vi "AlliGator Get Image Smoothing String.vi"(8 "Error In":errorcluster, 11 "Image Binning Options":T1 {"Bin" min=1}) -> (0 "Error Out":errorcluster, 3 "String":string)   [LabVIEW 2021, in "AlliGator Source Image.lvlib"]
doc: "Builds image smoothing options string."
uses:
  AlliGator Image Smoothing Options.ctl
  Arrays/Kernel Type.ctl
  Arrays/Smoothing Algorithm.ctl
  AlliGator Source Image.lvlib
  Arrays/Arrays.lvlib
  AlliGator Settings.lvlib
panel:
  # "see the AlliGator License on the block diagram (Ctrl+E or Window:Show Block Diagram)"
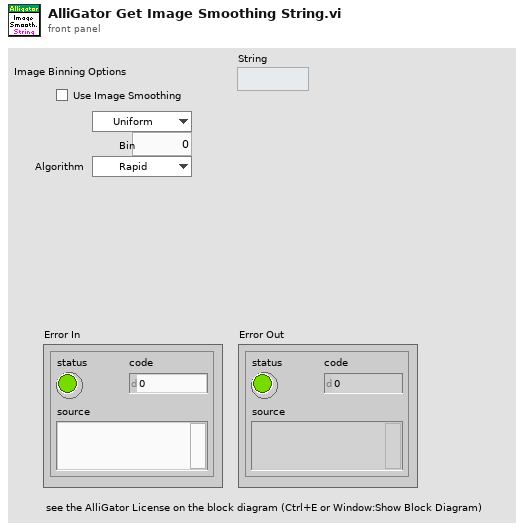
[diagram p1: front panel]
types:
  T1 = typedef "AlliGator Settings.lvlib/AlliGator Image Smoothing Options.ctl" = cluster{"Use Image Smoothing":bool, "Kernel Type":T2, "Bin":i32, "Algorithm":T3}
  T2 = typedef "Arrays.lvlib/Kernel Type.ctl" = enum16{"Uniform", "Bilinear", "Gaussian"}
  T3 = typedef "Arrays.lvlib/Smoothing Algorithm.ctl" = enum16{"Rapid", "Thorough"}
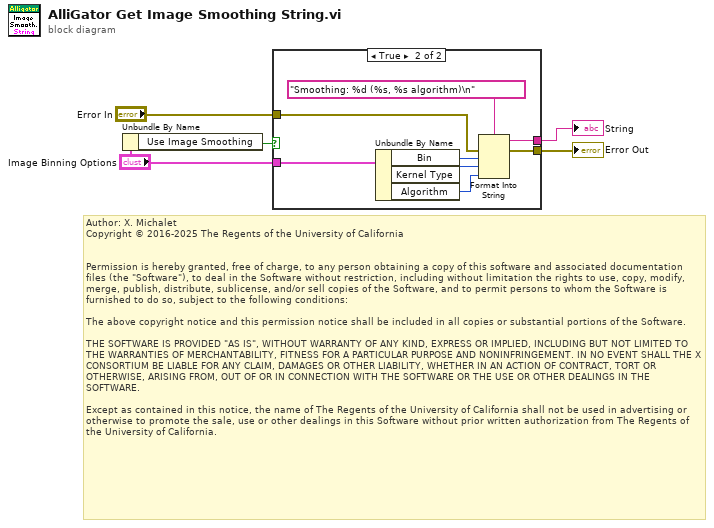
[diagram p0: block diagram]
diagram:
  # "Author: X. Michalet\nCopyright © 2016-2025 The Regents of the University of California\n \n\nPermission is hereby granted, free of charge, to any person obtaining a copy of this software and associated documentation files (the \"Software\"), to deal in the Software without restriction, including without limitation the rights to use, copy, modify, merge, publish, distribute, sublicense, and/or sell copies of the Software, and to permit persons to whom the Software is furnished to do so, subject to the following conditions:\n\nThe above copyright notice and this permission notice shall be included in all copies or substantial portions of the Software.\n\nTHE SOFTWARE IS PROVIDED \"AS IS\", WITHOUT WARRANTY OF ANY KIND, EXPRESS OR IMPLIED, INCLUDING BUT NOT LIMITED TO THE WARRANTIES OF MERCHANTABILITY, FITNESS FOR A PARTICULAR PURPOSE AND NONINFRINGEMENT. IN NO EVENT SHALL THE X CONSORTIUM BE LIABLE FOR ANY CLAIM, DAMAGES OR OTHER LIABILITY, WHETHER IN AN ACTION OF CONTRACT, TORT OR OTHERWISE, ARISING FROM, OUT OF OR IN CONNECTION WITH THE SOFTWARE OR THE USE OR OTHER DEALINGS IN THE SOFTWARE.\n\nExcept as contained in this notice, the name of The Regents of the University of California shall not be used in advertising or otherwise to promote the sale, use or other dealings in this Software without prior written authorization from The Regents of the University of California."
  n1 = Unbundle By Name("Image Binning Options") -> ("Use Image Smoothing"=w3:bool)
  n2 = case shown="True" w3 {
    tunnel: [_ w14] -> w5
    tunnel: "Image Binning Options" -> [_ w10]
    tunnel: "Error In" -> [w6 w13]
    tunnel: [w6 w12] -> w1
    frame False {
    }
    frame True {
      n3 = Unbundle By Name(w10) -> ("Bin"=w9:i32, "Kernel Type"=w8:T2, "Algorithm"=w7:T3)
      n4 = Format Into String(format string="Smoothing: %d (%s, %s algorithm)\n", error in=w13, w9, w8, w7) -> (resulting string=w14:string, error out=w12:errorcluster)  [unwired: 1 in]
    }
  }
  "String" <- w5
  "Error Out" <- w1
